vi "Sub 거리필터.vi"(8 "거리 데이터 열":i32, 9 "필터 거리(쉬프트 값보다 크게)":dbl, 10 "입력 배열(2차원)":dbl[][](array[numeric]), 11 "행 수":i32) -> (1 "거리필터된 갯수":i32, 3 "거리 필터된 배열":dbl[][](array[numeric]))   [LabVIEW 2016]
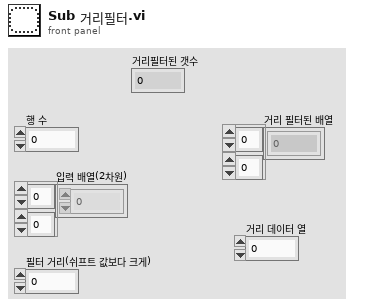
[diagram p1: front panel]
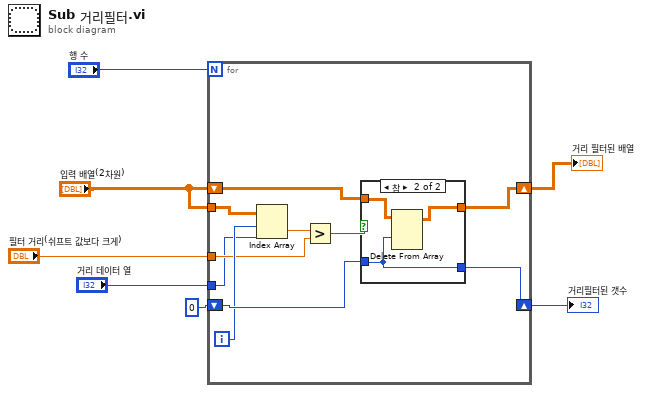
[diagram p0: block diagram]
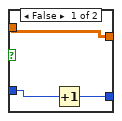
[diagram p2: hidden frame]
diagram:
  n1 = for {
    N: "행 수" -> [_]
    shift-right: [w13] -> w1
    shift-left: 0 ("비활성화된 인덱스 (열)") -> [w14]
    tunnel: "입력 배열(2차원)" -> [w15]
    shift-right: [w11] -> w4
    shift-left: "입력 배열(2차원)" -> [w12]
    tunnel: "필터 거리(쉬프트 값보다 크게)" -> [w9]
    tunnel: "거리 데이터 열" -> [w8]
    i -> [w10]
    n2 = Index Array(array=w15, index (row)=w10, index (col)=w8) -> (element=w17:dbl)
    n3 = Greater?(x=w17, y=w9) -> (0:w16:bool)
    n4 = case shown="참" w16 {
      tunnel: w14 -> [w20 w21]
      tunnel: [w18 w21] -> w13
      tunnel: [w19 w23] -> w11
      tunnel: w12 -> [w19 w22]
      frame False {
        n5 = Increment(x=w20) -> (x+1=w18:i32)
      }
      frame True {
        n6 = Delete From Array(array=w22, index (row)=w21) -> (array with subset deleted=w23:dbl[][])  [unwired: 2 in, 1 out]
      }
    }
  }
  "거리 필터된 배열" <- w4
  "거리필터된 갯수" <- w1
